vi "Is Clear.vi"(10 "Direction":T1, 11 "Maze":i32[](array[numeric])) -> (0 "Blocked?":bool, 1 "Can Move?":bool, 2 "Direction Out":T1, 3 "Maze":i32[](array[numeric]))   [LabVIEW 2015, in "Cross.lvclass"]
uses:
  Cross.lvclass
  Type Defs/Direction Enum.ctl
  SubVIs/Read-Only Globals.vi
  Square/Square.lvclass
  Type Defs/SB Type Defs.lvlib
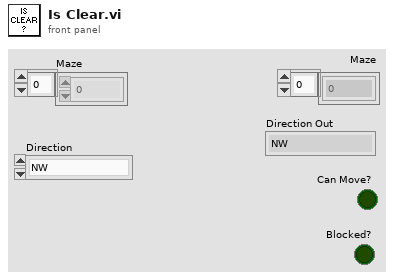
[diagram p1: front panel]
types:
  T1 = typedef "SB Type Defs.lvlib/Direction Enum.ctl" = enum16{"NW", "N", "NE", "E", "SE", "S", "SW", "W"}
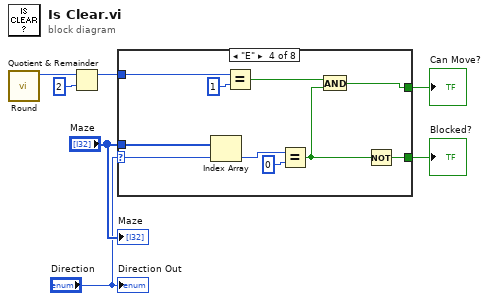
[diagram p0: block diagram]
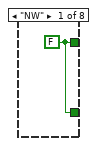
[diagram p2: hidden frame]
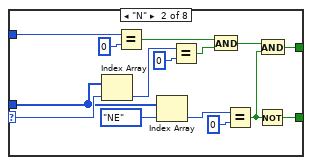
[diagram p3: hidden frame]
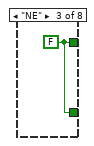
[diagram p4: hidden frame]
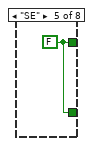
[diagram p5: hidden frame]
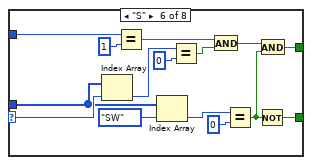
[diagram p6: hidden frame]
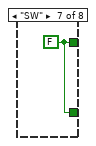
[diagram p7: hidden frame]
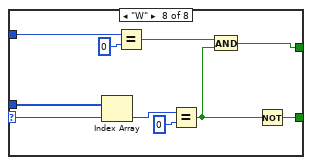
[diagram p8: hidden frame]
diagram:
  n1 = call "Round.vi"() -> ("Round"=w7:i32)  [unwired: 11 in]
  n2 = Quotient & Remainder(x=w7, y=2) -> (x-y*floor(x/y)=w5:i32)  [unwired: 1 out]
  n3 = case shown="\"E\"" "Direction" {
    selector: "Direction" -> [_ w18 _ w29 _ w44 _ w60]
    tunnel: w5 -> [_ w15 _ w30 _ w43 _ w58]
    tunnel: "Maze" -> [_ w17 _ w31 _ w42 _ w55]
    tunnel: [w8 w14 w24 w28 w35 w41 w51 w57] -> w3
    tunnel: [w8 w9 w24 w25 w35 w36 w51 w52] -> w1
    frame "NW" {
      w8 = FALSE
    }
    frame "N" {
      n4 = Index Array(array=w17, index=w18) -> (element=w22:i32)
      n5 = Equal?(x=w15, y=0) -> (x = y?=w11:bool)
      n6 = Index Array(array=w17, index=Direction_Enum."NE" ("Direction 2")) -> (element=w20:i32)
      n7 = Equal?(x=w22, y=0) -> (x = y?=w12:bool)
      n8 = And(x=w11, y=w12) -> (x .and. y?=w13:bool)
      n9 = Equal?(x=w20, y=0) -> (x = y?=w10:bool)
      n10 = Not(x=w10) -> (.not. x?=w9:bool)
      n11 = And(x=w13, y=w10) -> (x .and. y?=w14:bool)
    }
    frame "NE" {
      w24 = FALSE
    }
    frame "E" {
      n12 = Index Array(array=w31, index=w29) -> (element=w33:i32)
      n13 = Equal?(x=w30, y=1) -> (x = y?=w27:bool)
      n14 = Equal?(x=w33, y=0) -> (x = y?=w26:bool)
      n15 = And(x=w27, y=w26) -> (x .and. y?=w28:bool)
      n16 = Not(x=w26) -> (.not. x?=w25:bool)
    }
    frame "SE" {
      w35 = FALSE
    }
    frame "S" {
      n17 = Index Array(array=w42, index=w44) -> (element=w47:i32)
      n18 = Equal?(x=w43, y=1) -> (x = y?=w38:bool)
      n19 = Index Array(array=w42, index=Direction_Enum."SW" ("Direction 2")) -> (element=w49:i32)
      n20 = Equal?(x=w47, y=0) -> (x = y?=w39:bool)
      n21 = And(x=w38, y=w39) -> (x .and. y?=w40:bool)
      n22 = Equal?(x=w49, y=0) -> (x = y?=w37:bool)
      n23 = Not(x=w37) -> (.not. x?=w36:bool)
      n24 = And(x=w40, y=w37) -> (x .and. y?=w41:bool)
    }
    frame "SW" {
      w51 = FALSE
    }
    frame "W" {
      n25 = Index Array(array=w55, index=w60) -> (element=w56:i32)
      n26 = Equal?(x=w58, y=0) -> (x = y?=w54:bool)
      n27 = Equal?(x=w56, y=0) -> (x = y?=w53:bool)
      n28 = And(x=w54, y=w53) -> (x .and. y?=w57:bool)
      n29 = Not(x=w53) -> (.not. x?=w52:bool)
    }
  }
  "Can Move?" <- w3
  "Blocked?" <- w1
  "Maze" <- "Maze"
  "Direction Out" <- "Direction"
